vi "Panel Form Controller Config Constructor.vi"   [LabVIEW 2020, in "Panel Form Controller.lvlib"]
uses:
  Panel Form Controller.lvlib
  Form from Table Configuration/Form from Table Configuration.lvclass
  Form from Configured Table/Form from Configured Table.lvclass
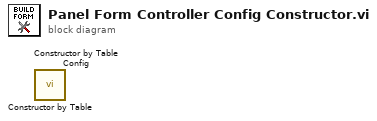
[diagram p0: block diagram]
diagram:
  n1 = call "Constructor by Table.vi"() -> ()  [unwired: 10 in, 2 out]
  n2 = call "Constructor by Table Config.vi"() -> ()  [unwired: 10 in, 2 out]
